vi "Initialise.vi"(8 "error in (no error)":errorcluster, 10 "System In":refnum<class "bt_System.lvclass">, 11 "Node in":refnum<class "bt_Blackboard Boolean Set.lvclass">) -> (0 "error out":errorcluster, 2 "System Out":refnum<class "bt_System.lvclass">, 3 "Node out":refnum<class "bt_Blackboard Boolean Set.lvclass">)   [LabVIEW 2021, in "BT.lvlib" / "bt_Blackboard Boolean Set.lvclass"]
uses:
  bt_Blackboard Boolean Set.lvclass
  bt_Blackboard Boolean Set.lvclass/bt_Blackboard Boolean Set.ctl
  Support/Nodes/Leaves/Blackboard/Type/bt_Blackboard_Leaf Type.lvclass
  Support/Blackboard/bt_Blackboard.lvclass
  Support/abs_System/bt_System.lvclass
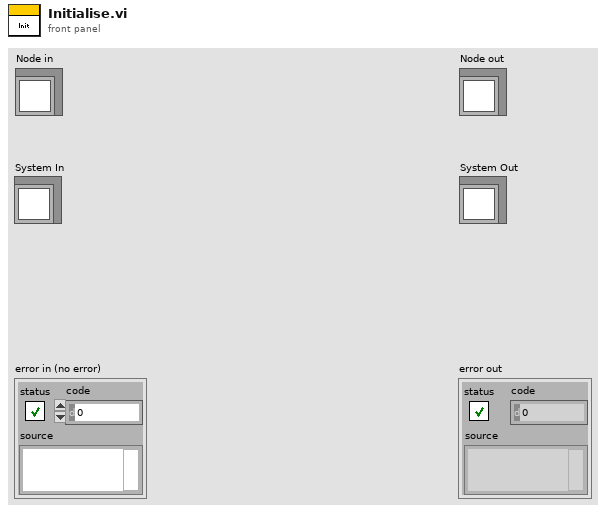
[diagram p1: front panel]
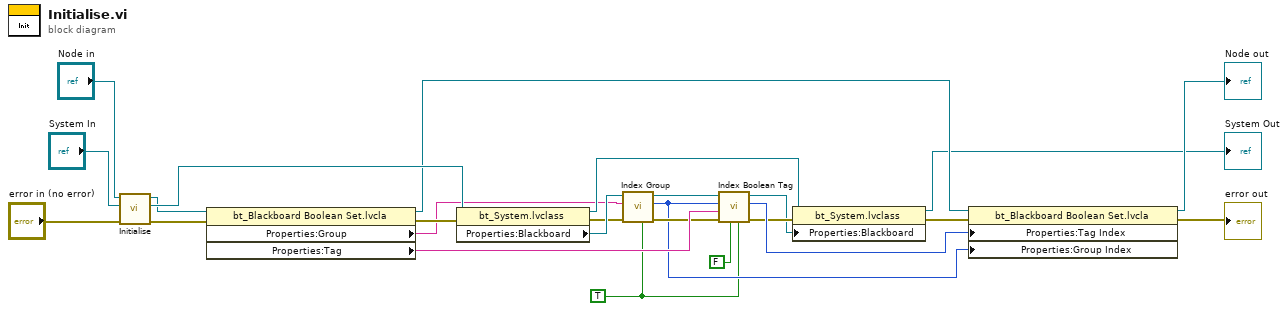
[diagram p0: block diagram]
diagram:
  w1 = TRUE ("Write?")
  n1 = call-parent "Initialise.vi"("error in (no error)"="error in (no error)", "System In"="System In", "Node in"="Node in") -> ("error out"=w21:errorcluster, "System Out"=w22:refnum<class "bt_System.lvclass">, "Node out"=w19:refnum<class "bt_Blackboard Boolean Set.lvclass">)  [unwired: 6 in]
  n2 = property class="bt_Blackboard Boolean Set.lvcla"(reference=w19, error in=w21) -> (reference out=w18:refnum<class "bt_Blackboard Boolean Set.lvclass">, error out=w20:errorcluster, "Properties:Group"=w3:string, "Properties:Tag"=w8:string)
  n3 = property class="bt_System.lvclass"(reference=w22, error in=w20) -> (reference out=w12:refnum<class "bt_System.lvclass">, error out=w4:errorcluster, "Properties:Blackboard"=w5:refnum<class "bt_Blackboard.lvclass">)
  n4 = call "Index Group.vi"("Write?"=w1, "error in (no error)"=w4, "Group"=w3, "bt_Blackboard in"=w5) -> ("error out"=w6:errorcluster, "Index"=w2:i32, "bt_Blackboard out"=w7:refnum<class "bt_Blackboard.lvclass">)  [unwired: 5 in]
  n5 = call "Index Boolean Tag.vi"("Write?"=w1, "Default Value"=FALSE, "error in (no error)"=w6, "Tag"=w8, "Group Index"=w2, "bt_Blackboard in"=w7) -> ("error out"=w14:errorcluster, "Index"=w15:i32, "bt_Blackboard out"=w13:refnum<class "bt_Blackboard.lvclass">)  [unwired: 2 in, 1 out]
  n6 = property class="bt_System.lvclass"(reference=w12, error in=w14, "Properties:Blackboard"=w13) -> (reference out=→"System Out":refnum<class "bt_System.lvclass">, error out=w10:errorcluster)
  n7 = property class="bt_Blackboard Boolean Set.lvcla"(reference=w18, error in=w10, "Properties:Tag Index"=w15, "Properties:Group Index"=w2) -> (reference out=→"Node out":refnum<class "bt_Blackboard Boolean Set.lvclass">, error out=→"error out":errorcluster)
